vi "Control Initialize.vi"(6 "Control Ref Cluster":T1, 8 "error in (no error)":errorcluster, 9 "Projection Palette Color":u32(colorbox), 10 "Ramp Palette Color":u32(colorbox), 11 "Main Frame Color":u32(colorbox)) -> (0 "error out":errorcluster, 1 "New Window Refnum":refnum<vi>)   [LabVIEW 2017, in "3D Plot.lvclass"]
uses:
  <vilib>/Math Plots/3D Math Plots/3D Plot/3D Plot/3D Plot.lvclass
  <vilib>/Math Plots/3D Math Plots/3D Plot/Action String/3DMathPlot Ctrl Act Cluster.ctl
  <vilib>/Math Plots/3D Math Plots/3D Plot/Action String/3DMathPlot State Class.ctl
  <vilib>/picture/3D Picture Control/NI_3D Picture Control.lvlib
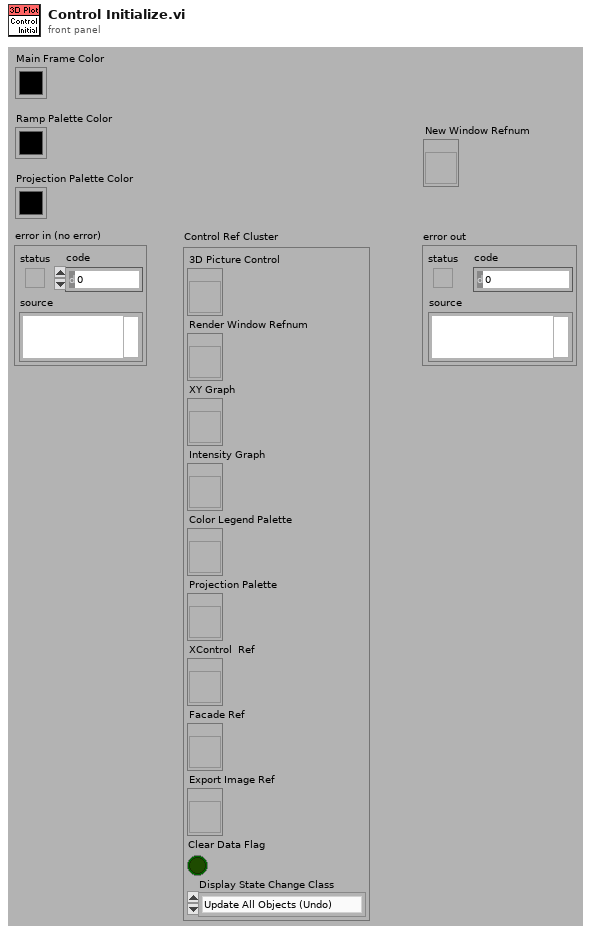
[diagram p1: front panel]
types:
  T1 = typedef "3DMathPlot Ctrl Act Cluster.ctl" = cluster{"3D Picture Control":refnum<vi>, "Render Window Refnum":refnum<vi>, "XY Graph":refnum<vi>, "Intensity Graph":refnum<vi>, "Color Legend Palette":refnum<vi>, "Projection Palette":refnum<vi>, "XControl  Ref":refnum<vi>, "Facade Ref":refnum<vi>, "Export Image Ref":refnum<vi>, "Clear Data Flag":bool, "Display State Change Class":T2}
  T2 = typedef "3DMathPlot State Class.ctl" = enum16{"Update All Objects (Undo)", "Update Light Object Only", "Update Axis Object Only", "Update Plot Object Only", "Update Cursor Object Only", "Update Axis Plot Cursor Objects", "No Update"}
  T3 = enum16{"Open", "Minimized", "Maximized", "Hidden"}
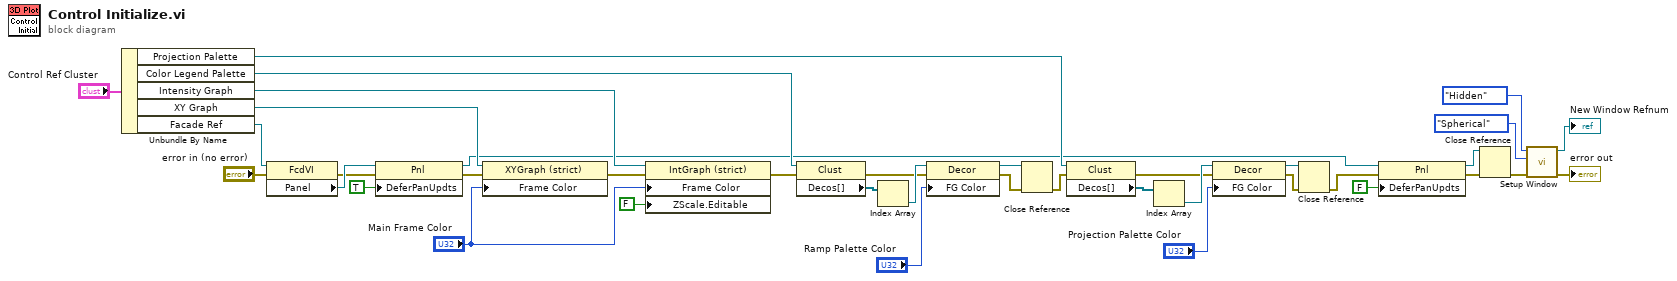
[diagram p0: block diagram]
diagram:
  n1 = Unbundle By Name("Control Ref Cluster") -> ("Projection Palette"=w19:refnum<vi>, "Color Legend Palette"=w20:refnum<vi>, "Intensity Graph"=w21:refnum<vi>, "XY Graph"=w22:refnum<vi>, "Facade Ref"=w10:refnum<vi>)
  n2 = property class="FcdVI"(reference=w10, error in="error in (no error)") -> (error out=w13:errorcluster, "Panel"=w18:refnum<vi>)  [unwired: 1 out]
  n3 = property class="Pnl"(reference=w18, error in=w13, "DeferPanUpdts"=TRUE ("Defer Panel Updates")) -> (reference out=w15:refnum<vi>, error out=w12:errorcluster)
  n4 = property class="XYGraph (strict)"(reference=w22, error in=w12, "Frame Color"="Main Frame Color") -> (error out=w27:errorcluster)  [unwired: 1 out]
  n5 = property class="IntGraph (strict)"(reference=w21, error in=w27, "Frame Color"="Main Frame Color", "ZScale.Editable"=FALSE ("Z Scale.Editable")) -> (error out=w26:errorcluster)  [unwired: 1 out]
  n6 = property class="Clust"(reference=w20, error in=w26) -> (error out=w25:errorcluster, "Decos[]"=w33:refnum<vi>[])  [unwired: 1 out]
  n7 = Index Array(array=w33) -> (element=w32:refnum<vi>)  [unwired: 1 in]
  n8 = property class="Decor"(reference=w32, error in=w25, "FG Color"="Ramp Palette Color") -> (reference out=w6:refnum<vi>, error out=w4:errorcluster)
  n9 = Close Reference(reference=w6, error in (no error)=w4) -> (error out=w3:errorcluster)
  n10 = property class="Clust"(reference=w19, error in=w3) -> (error out=w24:errorcluster, "Decos[]"=w29:refnum<vi>[])  [unwired: 1 out]
  n11 = Index Array(array=w29) -> (element=w30:refnum<vi>)  [unwired: 1 in]
  n12 = property class="Decor"(reference=w30, error in=w24, "FG Color"="Projection Palette Color") -> (reference out=w5:refnum<vi>, error out=w2:errorcluster)
  n13 = Close Reference(reference=w5, error in (no error)=w2) -> (error out=w1:errorcluster)
  n14 = property class="Pnl"(reference=w15, error in=w1, "DeferPanUpdts"=FALSE ("Defer Panel Updates")) -> (reference out=w9:refnum<vi>, error out=w8:errorcluster)
  n15 = Close Reference(reference=w9, error in (no error)=w8) -> (error out=w7:errorcluster)
  n16 = call <vilib>:"Setup Window.vi"("error in (no error)"=w7, "Camera Controller"=enum16{"None", "Spherical", "Flying"}."Spherical", "Window State"=T3."Hidden") -> ("error out"=→"error out":errorcluster, "New Window Refnum"=→"New Window Refnum":refnum<vi>)  [unwired: 7 out]
